vi "Temp Deg C to F.vi"() -> ()   [LabVIEW 2023]
panel:
  out "Temp (Deg F)":dbl
  in  "Temp (Deg C)":dbl
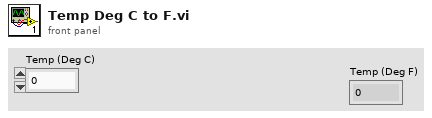
[diagram p1: front panel]
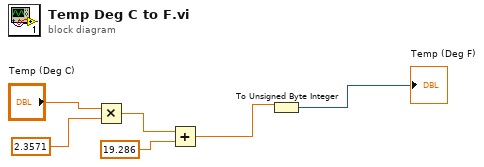
[diagram p0: block diagram]
diagram:
  n1 = Multiply(x="Temp (Deg C)", y=2.3571) -> (x*y=w4:dbl)
  n2 = Add(x=w4, y=19.286) -> (x+y=w2:dbl)
  n3 = To Unsigned Byte Integer(number=w2) -> (unsigned 8bit integer=→"Temp (Deg F)":u8)
